vi "Manual Test.vi"() -> ()   [LabVIEW 2020, in "ChromTech Series III Pump.lvlib"]
uses:
  <instrlib>/RxnRover/ChromtechSeriesIIIDriver/ChromTech Series III Pump.lvlib
panel:
  out "error out":errorcluster
  in  "Stop Pump":bool
  in  "Start Pump":bool
  in  "Get User Compensation":bool
  out "Current User Compensation":dbl
  in  "stop":bool
  in  "error in (no error)":errorcluster
  in  "Get Current Status":bool
  out "Pressure Units":string
  out "Lower Pressure Limit":dbl
  out "Upper Pressure Limit":dbl
  in  "Get Pump Information":bool
  out "Lower Pressure Fault":bool
  out "Motor Stall":bool
  out "Keypad Enabled":bool
  out "Upper Pressure Fault":bool
  out "In Prime":bool
  out "Running":bool
  out "Head Identifier":string
  out "Pressure Compensation":i32
  out "Current Flow Rate":dbl
  out "Current Pressure":dbl
  in  "Get Current Conditions":bool
  in  "Get Firmware Details":bool
  out "Firmware Version":dbl
  in  "Set User Comp":bool
  in  "Pressure Compensation":dbl=100.0
  in  "VISA resource name":refnum<visa-resource-name>
  in  "Set Flow Rate":bool
  in  "Flow Rate":dbl
  # "ChromTech Series III Pump"
  # "Set Conditions"
  # "Current Status"
  # "Firmware Information"
  # "Still Under constuction. Should probably be reworked into state machine and \nexplicitly make a test button for each driver VI."
  # "This is currently broken and needs to be rewritten!"
  # "Get Conditions"
  # "Pump Information"
  # "Pump Control"
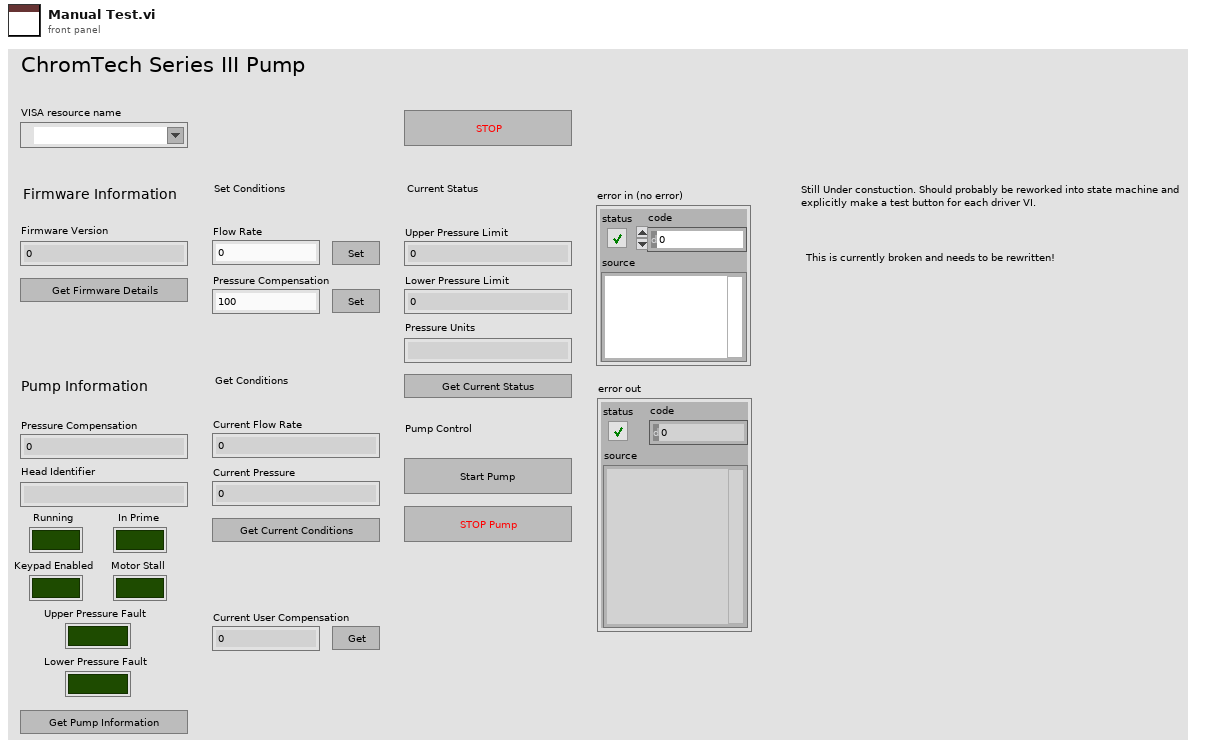
[diagram p1: front panel]
types:
  T1 = cluster{"Baud Rate":u32, "Parity":u16, "Flow Control":u16, "Data Bits":u16, "Stop Bits":u16}
  T2 = cluster{"Flow rate":dbl, "Running":bool, "Pressure Comp":i32, "Head Type":i32, "Upper Pressure Fault":bool, "Lower Pressure Fault":bool, "In Prime":bool, "Keypad Enabled":bool, "Motor Stall Fault":bool, "Pressure Board present":bool, "External control mode":i32, "Started and frequency controlled":bool, "Started and voltage controlled":bool, "PUMP-RUN input":bool, "PUMP-STOP input":bool, "ENABLE IN input":bool}
  T3 = cluster{"Flow rate":dbl, "Upper Pressure Limit":dbl, "Lower Pressure Limit":dbl, "Pressure Units":string, "Running?":bool, "Pressure Board Present?":bool, "Macro Pump Head?":bool}
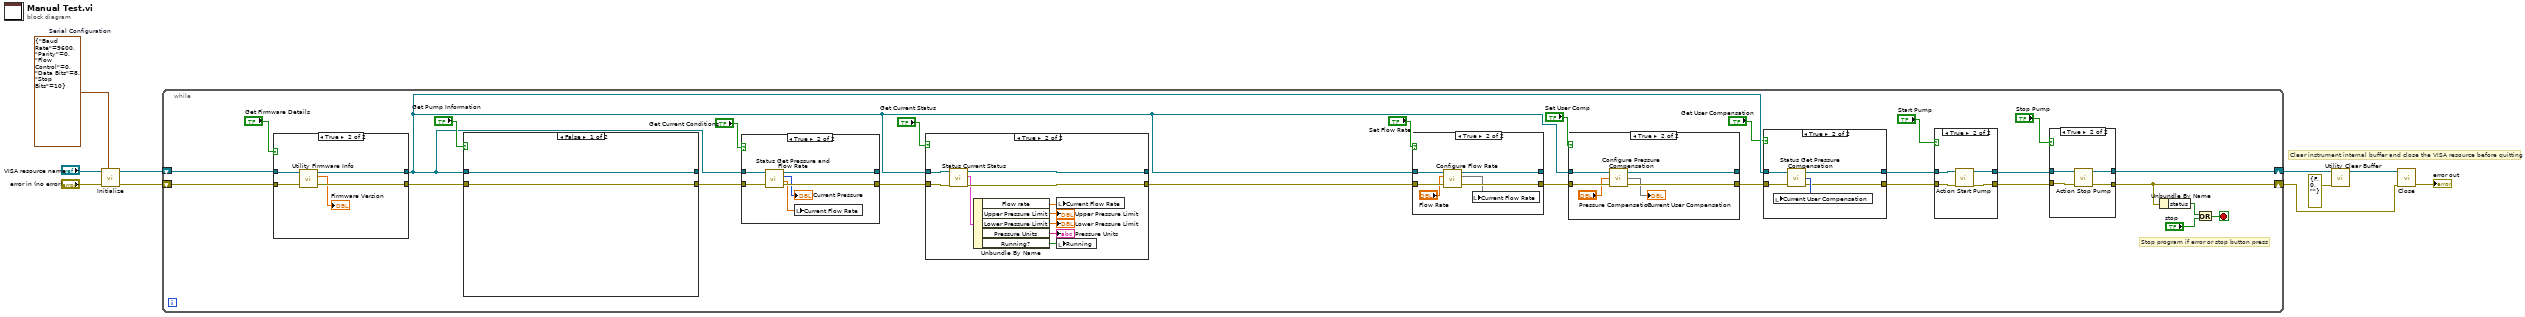
[diagram p0: block diagram]
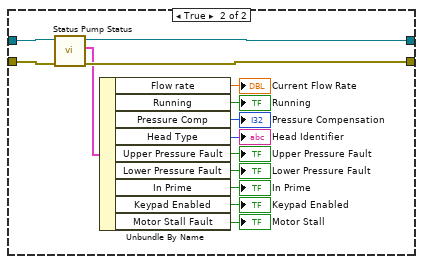
[diagram p9: hidden frame]
diagram:
  w6 = T1 {"Baud Rate"=9600, "Parity"=0, "Flow Control"=0, "Data Bits"=8, "Stop Bits"=10}  # Serial Configuration
  # "Clear instrument internal buffer and close the VISA resource before quitting"
  n1 = call <instrlib>:"Initialize.vi"("Serial Configuration"=w6, "error in (no error)"="error in (no error)", "VISA resource name"="VISA resource name") -> ("error out"=w7:errorcluster, "VISA resource name out"=w9:refnum<visa-resource-name>)  [unwired: 7 in]
  n2 = while {
    shift-right: [w11] -> w1
    shift-left: w7 -> [w36]
    shift-right: [w12] -> w3
    shift-left: w9 -> [w28]
    stop <- w15 stop-if-true
    # "Stop program if error or stop button press"
    n3 = case shown="True" "Get Firmware Details" {
      tunnel: w28 -> [w108 w113]
      tunnel: w36 -> [w107 w112]
      tunnel: [w108 w111] -> w30
      tunnel: [w107 w110] -> w27
      frame False {
      }
      frame True {
        n4 = call <instrlib>:"Utility Firmware Info.vi"("error in"=w112, "VISA resource name"=w113) -> ("error out"=w110:errorcluster, "Firmware Version"=→"Firmware Version":dbl, "VISA resource name out"=w111:refnum<visa-resource-name>)  [unwired: 7 in]
      }
    }
    n5 = case shown="False" "Get Pump Information" {
      tunnel: w30 -> [w93 w106]
      tunnel: [w93 w105] -> _
      tunnel: w27 -> [w92 w104]
      tunnel: [w92 w104] -> w26
      frame False {
      }
      frame True {
        n6 = call <instrlib>:"Status Pump Status.vi"("error in (no error)"=w104, "VISA resource name"=w106) -> ("Status Cluster"=w103:T2, "VISA resource name out"=w105:refnum<visa-resource-name>)  [unwired: 7 in, 1 out]
        n7 = Unbundle By Name(w103) -> ("Flow rate"=→"Current Flow Rate":dbl, "Running"=→"Running":bool, "Pressure Comp"=→"Pressure Compensation":i32, "Head Type"=→"Head Identifier":i32, "Upper Pressure Fault"=→"Upper Pressure Fault":bool, "Lower Pressure Fault"=→"Lower Pressure Fault":bool, "In Prime"=→"In Prime":bool, "Keypad Enabled"=→"Keypad Enabled":bool, "Motor Stall Fault"=→"Motor Stall":bool)
      }
    }
    n8 = case shown="True" "Get Current Conditions" {
      tunnel: w30 -> [w85 w91]
      tunnel: [w85 w90] -> _
      tunnel: w26 -> [w84 w89]
      tunnel: [w84 w88] -> w25
      frame False {
      }
      frame True {
        n9 = call <instrlib>:"Status Get Pressure and Flow Rate.vi"("error in"=w89, "VISA resource name"=w91) -> ("error out"=w88:errorcluster, "Flow Rate"=w86:dbl, "Pressure"=→"Current Pressure":i32, "VISA resource name out"=w90:refnum<visa-resource-name>)  [unwired: 6 in]
        n10 = local write "Current Flow Rate"(w86) -> ()
      }
    }
    n11 = case shown="True" "Get Current Status" {
      tunnel: w30 -> [w72 w83]
      tunnel: [w72 w82] -> _
      tunnel: w25 -> [w73 w81]
      tunnel: [w73 w80] -> w24
      frame False {
      }
      frame True {
        n12 = call <instrlib>:"Status Current Status.vi"("error in (no error)"=w81, "VISA resource name"=w83) -> ("error out"=w80:errorcluster, "Status Cluster"=w79:T3, "VISA resource name out"=w82:refnum<visa-resource-name>)  [unwired: 7 in]
        n13 = Unbundle By Name(w79) -> ("Flow rate"=w78:dbl, "Upper Pressure Limit"=→"Upper Pressure Limit":dbl, "Lower Pressure Limit"=→"Lower Pressure Limit":dbl, "Pressure Units"=→"Pressure Units":string, "Running?"=w74:bool)
        n14 = local write "Current Flow Rate"(w78) -> ()
        n15 = local write "Running"(w74) -> ()
      }
    }
    n16 = case shown="True" "Set Flow Rate" {
      tunnel: w30 -> [w65 w71]
      tunnel: w24 -> [w64 w69]
      tunnel: [w65 w70] -> _
      tunnel: [w64 w68] -> w23
      frame False {
      }
      frame True {
        n17 = call <instrlib>:"Configure Flow Rate.vi"("error in"=w69, "Flow Input (ml/min)"="Flow Rate", "VISA resource name"=w71) -> ("error out"=w68:errorcluster, 2:w66, "VISA resource name out"=w70:refnum<visa-resource-name>)  [unwired: 6 in]
        n18 = local write "Current Flow Rate"(w66) -> ()
      }
    }
    n19 = case shown="True" "Set User Comp" {
      tunnel: w30 -> [w58 w63]
      tunnel: w23 -> [w57 w61]
      tunnel: [w58 w62] -> _
      tunnel: [w57 w61] -> w22
      frame False {
      }
      frame True {
        n20 = call <instrlib>:"Configure Pressure Compensation.vi"("error in"=w61, "Pressure Compensation (PSI)"="Pressure Compensation", "VISA resource name"=w63) -> (1:→"Current User Compensation", "VISA resource name out"=w62:refnum<visa-resource-name>)  [unwired: 1 out]
      }
    }
    n21 = case shown="True" "Get User Compensation" {
      tunnel: w30 -> [w51 w56]
      tunnel: w22 -> [w50 w54]
      tunnel: [w50 w52] -> w19
      tunnel: [w51 w55] -> w20
      frame False {
      }
      frame True {
        n22 = call <instrlib>:"Status Get Pressure Compensation.vi"("error in"=w54, "VISA resource name"=w56) -> ("error out"=w52:errorcluster, "User Compensation"=w53:i32, "VISA resource name out"=w55:refnum<visa-resource-name>)  [unwired: 1 in]
        n23 = local write "Current User Compensation"(w53) -> ()
      }
    }
    n24 = case shown="True" "Start Pump" {
      tunnel: [w45 w47] -> w17
      tunnel: w20 -> [w45 w48]
      tunnel: [w44 w46] -> w16
      tunnel: w19 -> [w44 w49]
      frame False {
      }
      frame True {
        n25 = call <instrlib>:"Action Start Pump.vi"("error in"=w49, "VISA resource name"=w48) -> ("error out"=w46:errorcluster, "VISA resource name out"=w47:refnum<visa-resource-name>)  [unwired: 8 in]
      }
    }
    n26 = case shown="True" "Stop Pump" {
      tunnel: [w39 w41] -> w12
      tunnel: w17 -> [w39 w42]
      tunnel: [w38 w40] -> w11
      tunnel: w16 -> [w38 w43]
      frame False {
      }
      frame True {
        n27 = call <instrlib>:"Action Stop Pump.vi"("error in"=w43, "VISA resource name"=w42) -> ("error out"=w40:errorcluster, "VISA resource name out"=w41:refnum<visa-resource-name>)  [unwired: 8 in]
      }
    }
    n28 = Unbundle By Name(w11) -> ("status"=w14:bool)
    n29 = Or(x=w14, y="stop") -> (x .or. y?=w15:bool)
  }
  n30 = call <instrlib>:"Utility Clear Buffer.vi"("error in (no error)"=errorcluster {"status"=FALSE, "code"=0, "source"=""}, "VISA resource name"=w3) -> ("VISA resource name out"=w5:refnum<visa-resource-name>)  [unwired: 8 in, 1 out]
  n31 = call <instrlib>:"Close.vi"("error in (no error)"=w1, "VISA resource name"=w5) -> ("error out"=→"error out":errorcluster)  [unwired: 9 in]
